vi "GitLoad.vi"(7 "Viewer?":bool, 8 "error in (no error)":errorcluster, 9 "Directory":path=path "", 10 "LoadThisHash":string, 11 "Git exec":string="git") -> (0 "error out":errorcluster, 1 "Directory out":path, 2 "Save Cluster":T1={"Version"="", "Devices"=[], "Select Layout"=0, "Layout:Strings And Values []"=[], "User defined functions"="-- -------------------------------------------------------------------------------------------\n-- The following functions are part of the \"standard load\" of functions and should not be messed with\n-- They are here for reference only.\n-- Please add any user functions above this comment\n-- -------------------------------------------------------------------------------------------\n\n-- Creates a linear ramp from A to B\nfunction LineRamp(f, Initial, Final)\n    return (1-f)*Initial + f*Final;\nend\n\n-- Creates an exponential ramp from A to B\nfunction ExpRamp(t, a, b, tau)\n   return (b - a*exp(tMax / tau) + (a-b)*exp(t/tau))/ ( 1 - exp(tMax / tau) );\nend\n\n-- Creates a sinewave\nfunction SinRamp(t,Offset,A,Freq, Phase)\n    return Offset + A * sin(2*pi*Freq*t + Phase)\nend\n\n-- Creates a blackman pulse\nfunction Blackman(f, Offset, A)\n    return Offset +  A*sqrt(0.5*cos(3.1415*(2*f-1))+0.08*cos(2*pi*(2*f-1))+0.42);\nend\n\n-- Creates a half-gauss ramp\nfunction HalfGaussRamp(t, a, b, Width)\n    local y;\n    y = exp(-(tMax^2)/Width^2);\n    y = (a -  b*y)/(1-y)  +  ((b-a)/(1-y))*exp(-((t-tMax)^2)/Width^2);\n    return y;\nend\n\n-- Creates an \"O'Hara\" ramp from A to B, for dipole evaporation\nfunction EvapRamp(t, a, b, tau)\n   local y;\n  y = log(a/b) / log(1+tMax/tau);\n  y = a * (1+t/tau)^(-y);\n  return y;\nend\n", "VariableManager"=refnum} {"Select Layout" items=["Default"]}, 3 "Git exec out":string, 4 "Loaded Description":string, 5 "User Cancelled":bool, 6 "Loaded Commit Info":T3)   [LabVIEW 2013]
uses:
  GitCommitCluster/CommitCluster.ctl
  TypeDefs/SaveCluster.ctl
  VariableManagerCodes/VariableManager/VariableManager.lvclass
  DeviceVIs/Device/Device.lvclass
  <vilib>/Utility/miscctls.llb/LVStringsAndValuesArrayTypeDef_I32.ctl
  <vilib>/Utility/miscctls.llb/LVPointTypeDef.ctl
  <vilib>/Utility/error.llb/DialogType.ctl
  <vilib>/Utility/miscctls.llb/LVRowAndColumnUnsignedTypeDef.ctl
panel:
  in  "WhichLoad":enum32{"Simple", "Filter"}(tab)
  in  "LoadSimple":bool
  in  "Page":u32=1 caption="Page (of 3)" min=1 max=3 step=1
  in  "SimpleProcedure":i32(listbox) caption="Pick a Procedure"
  in  "Cancel Button":bool
  in  "ToFilter":bool
  in  "CaseSensitive?":bool
  in  "MatchAll?":bool
  in  "Patterns":string[][](table)
  in  "AuthorList":i32[](listbox)
  out "Number Matched":i32
  in  "ApplyFilter":bool
  in  "AfterFilter":timestamp format="%<%H:%M:%S\n%Y/%m/%d>T"
  in  "BeforeFilter":timestamp format="%<%H:%M:%S\n%Y/%m/%d>T"
  in  "AfterDate?":bool
  in  "HashFilter":u64 format="%x"
  in  "Description?":bool
  in  "Author?":bool
  in  "BeforeDate?":bool
  in  "Hash?":bool
  in  "Cancel Button 2":bool
  in  "LoadFiltered":bool
  in  "ToSimple":bool
  in  "FilterProcedure":i32(listbox) caption="Pick a Procedure"
  # "Note: Sorting only affects entries on this page"
  # "(Uses grep-style expressions)"
  # "These are commit dates, which may be different from the \"date\" column."
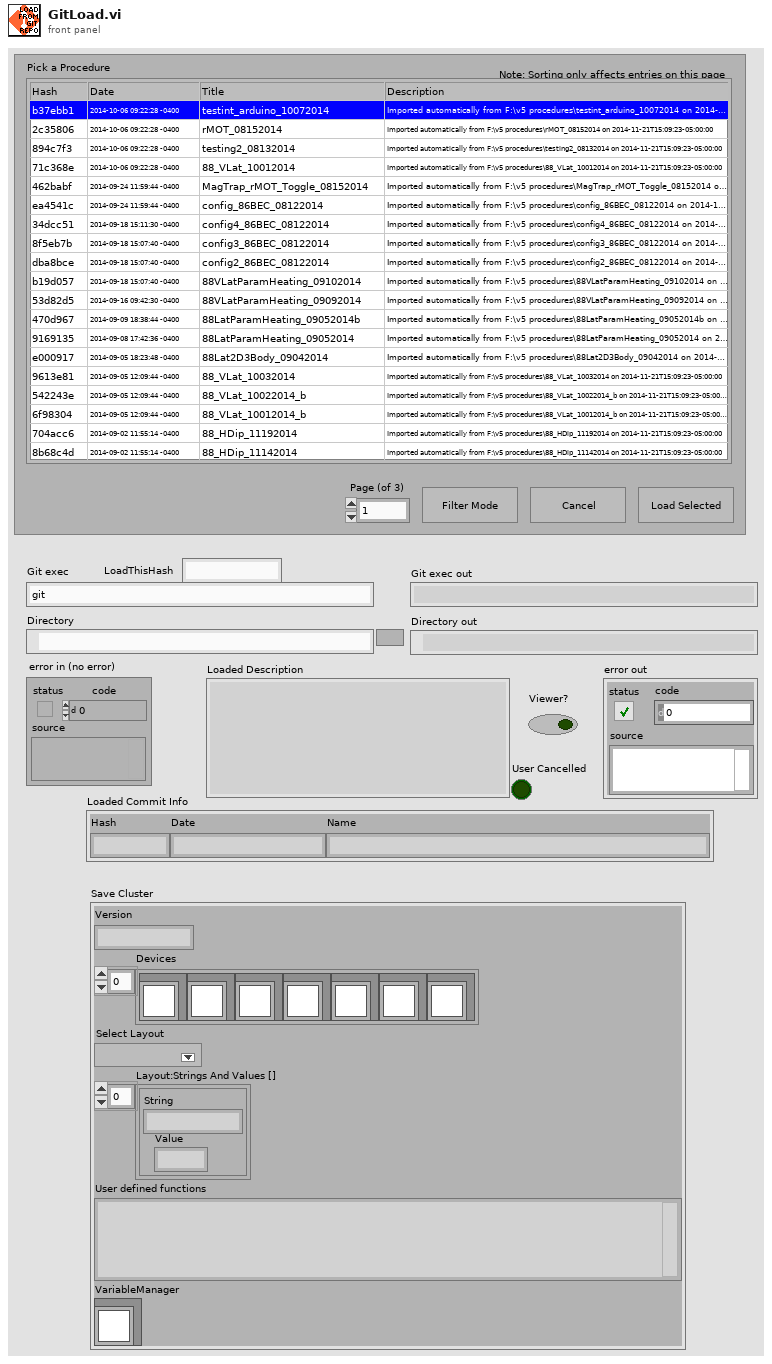
[diagram p1: front panel]
types:
  T1 = typedef "SaveCluster.ctl" = cluster{"Version":string, "Devices":refnum<class "Device.lvclass">[], "Select Layout":i32, "Layout:Strings And Values []":T2, "User defined functions":string, "VariableManager":refnum<class "VariableManager.lvclass">}
  T2 = typedef "LVStringsAndValuesArrayTypeDef_I32.ctl" = cluster{"String":string, "Value":i32}[]
  T3 = typedef "CommitCluster.ctl" = cluster{"Hash":string, "Date":string, "Name":string}
  T4 = typedef "DialogType.ctl" = u16
  T5 = typedef "LVPointTypeDef.ctl" = cluster{"Horizontal":i16, "Vertical":i16}
  T6 = typedef "LVRowAndColumnUnsignedTypeDef.ctl" = cluster{"Row":u32, "Column":u32}
  T7 = cluster{"Hash?":bool, "HashFilter":u64, "Description?":bool, "DescTitleFilters":string[], "MatchAll?":bool, "AfterDate?":bool, "AfterFilter":timestamp, "BeforeDate?":bool, "BeforeFilter":timestamp, "Author?":bool, "AuthorList":string[], "SelectedAuthors":i32[], "CaseSensitive?":bool}
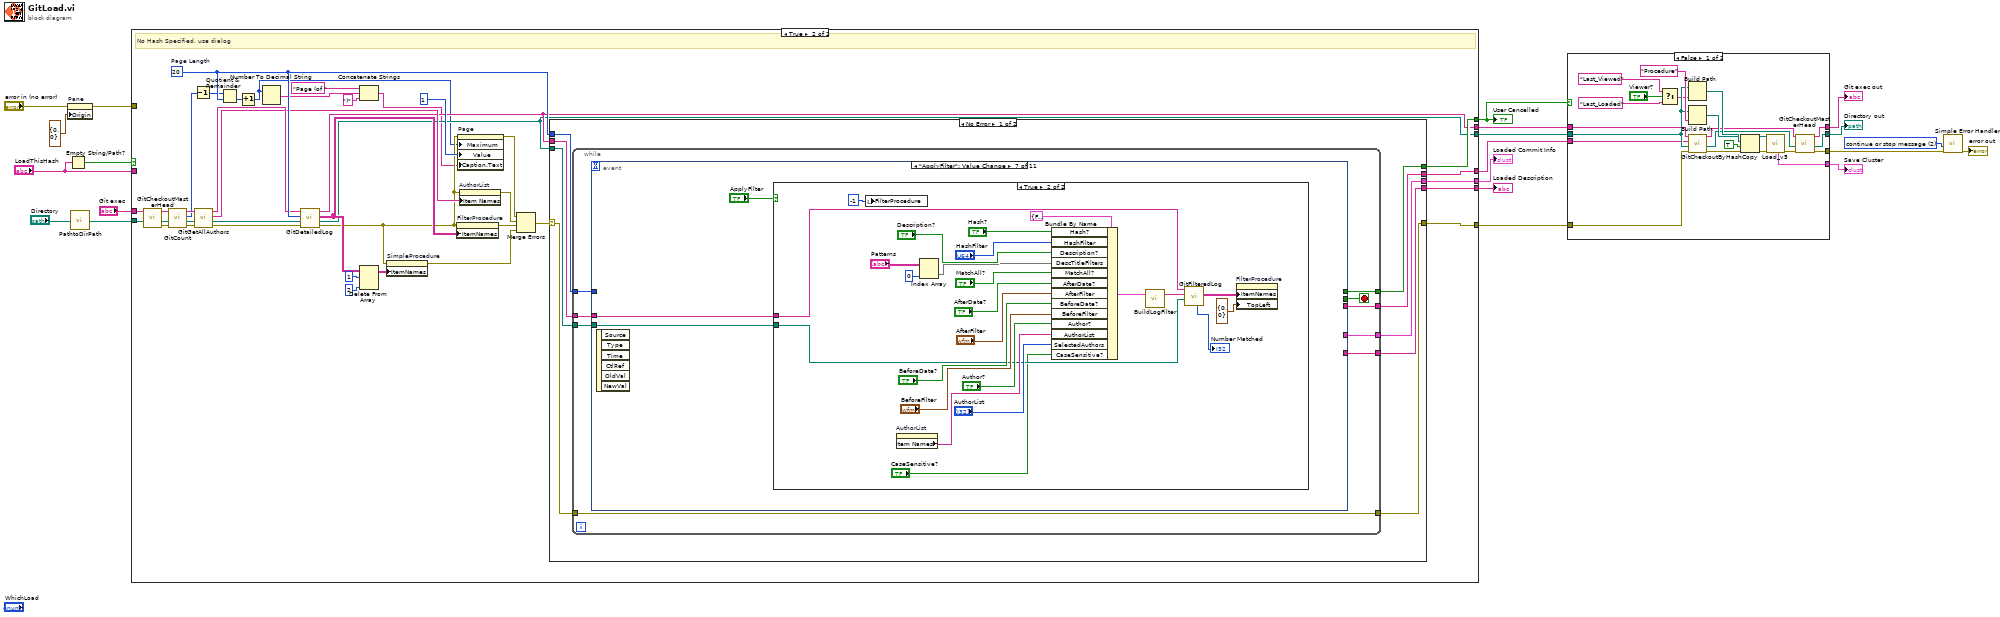
[diagram p0: block diagram]
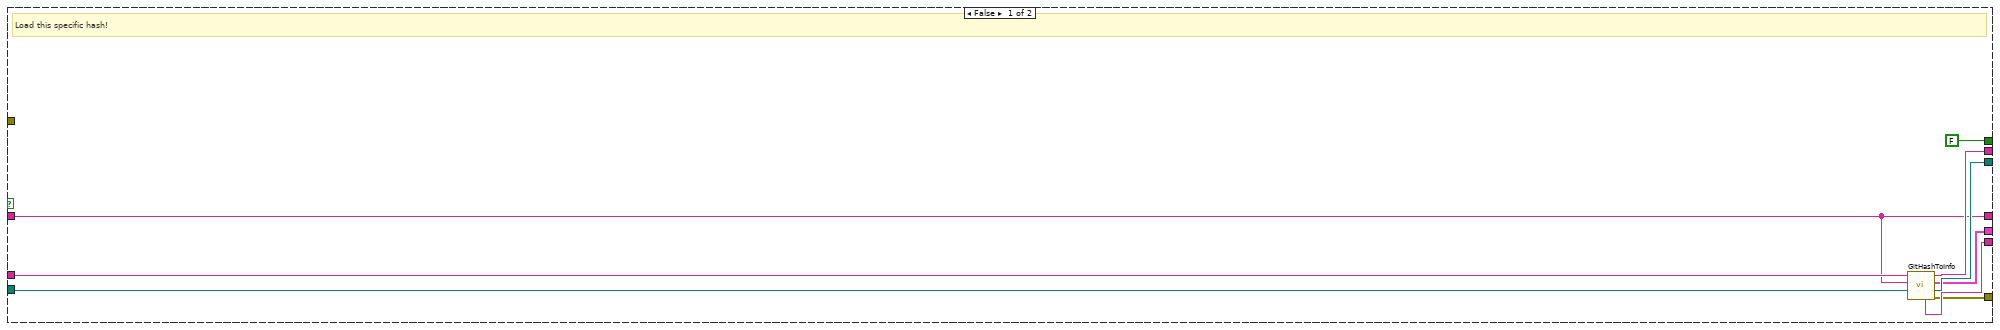
[diagram p2: hidden frame]
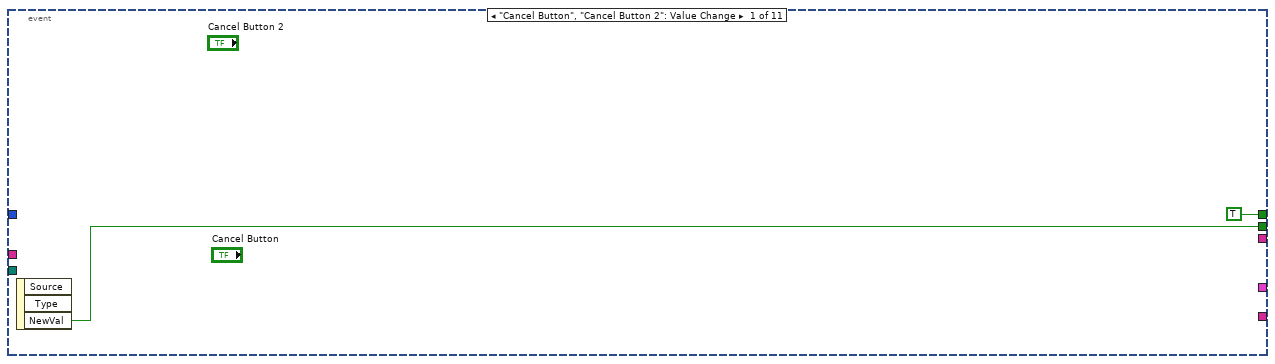
[diagram p3: hidden frame]
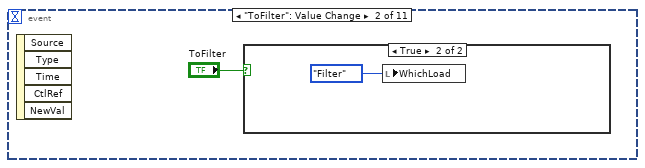
[diagram p4: hidden frame]
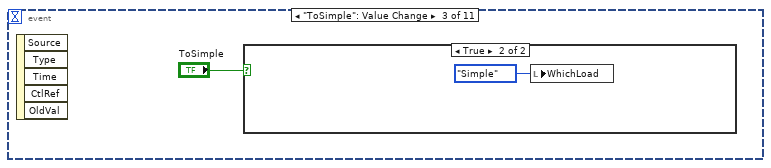
[diagram p6: hidden frame]
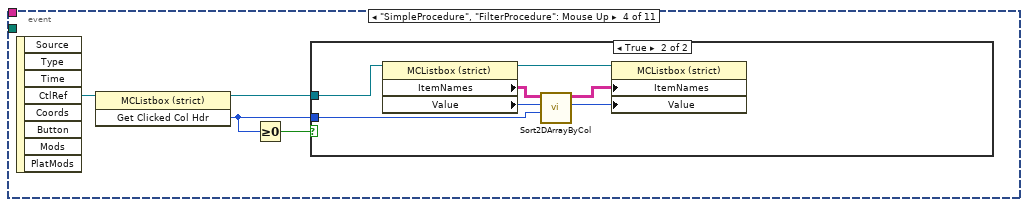
[diagram p8: hidden frame]
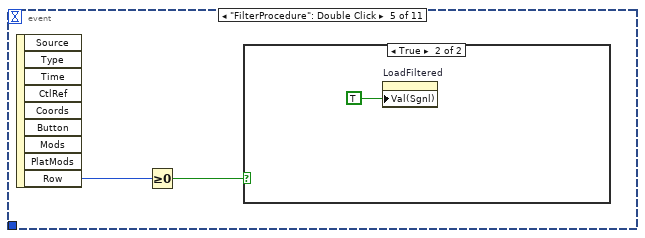
[diagram p10: hidden frame]
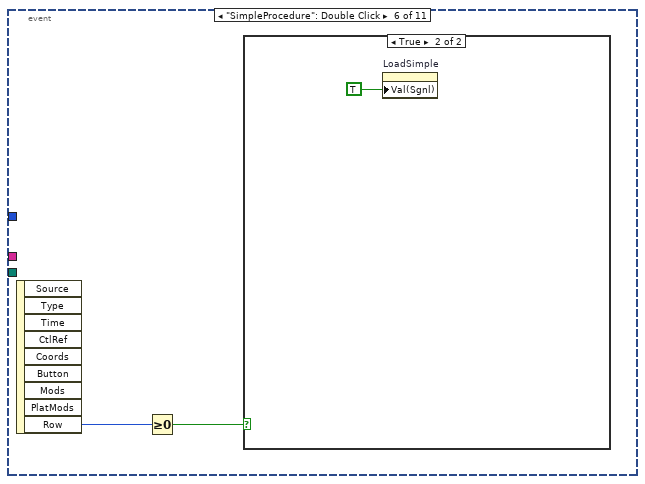
[diagram p12: hidden frame]
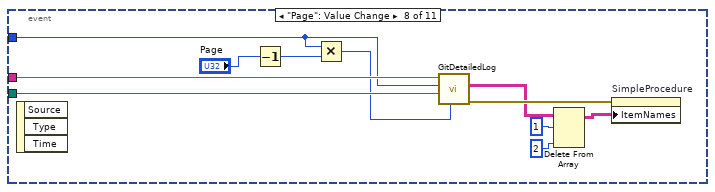
[diagram p15: hidden frame]
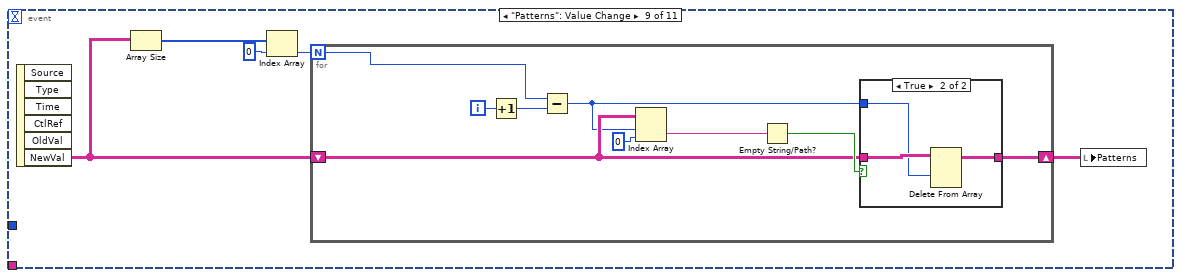
[diagram p16: hidden frame]
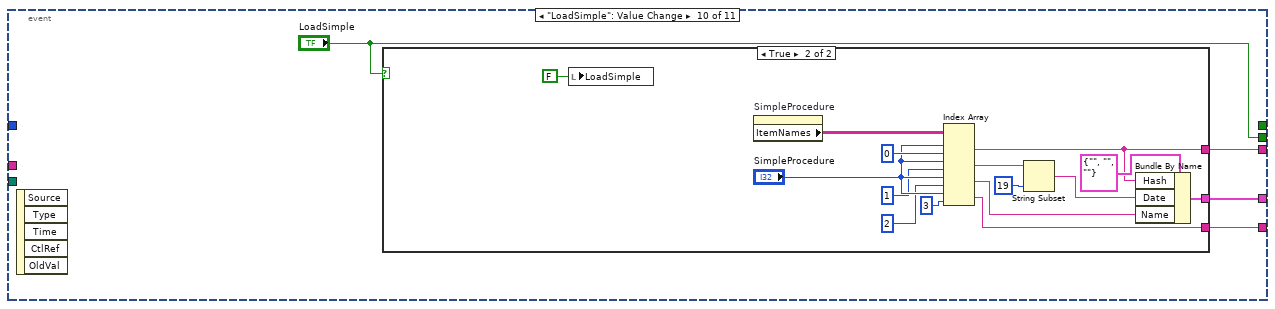
[diagram p18: hidden frame]
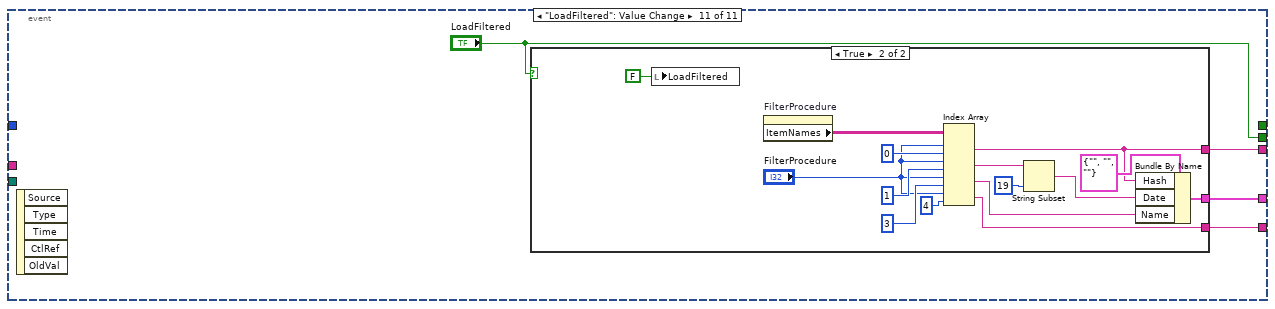
[diagram p20: hidden frame]
diagram:
  w3 = T4 2 items=["no dialog", "OK message", "continue or stop message", "OK message + warnings", "continue/stop + warnings"] ("type of dialog (OK msg:1)")
  n1 = property on="Pane" class="Pane"(error in="error in (no error)", "Origin"=T5 {"Horizontal"=0, "Vertical"=0}) -> (error out=w4:errorcluster)  [unwired: 1 in, 1 out]
  n2 = Empty String/Path?(string/path="LoadThisHash") -> (empty?=w6:bool)
  n3 = call "PathtoDirPath.vi"("Path"="Directory") -> ("Path out"=w15:path)
  n4 = case shown="True" w6 {
    tunnel: [w22 w56] -> w21
    tunnel: [FALSE w55] -> w20
    tunnel: [w28 w54] -> w19
    tunnel: [w29 w53] -> w18
    tunnel: "Git exec" -> [w27 w49]
    tunnel: w15 -> [w26 w48]
    tunnel: [w25 w47] -> w12
    tunnel: [w24 w46] -> w11
    tunnel: [w23 w39] -> w10
    tunnel: "LoadThisHash" -> [w22 _]
    tunnel: w4 -> [_ _]
    frame False {
      # "Load this specific hash!"
      n5 = call "GitHashToInfo.vi"("Directory"=w26, "Hash"=w22, "Git exec"=w27) -> ("error out"=w23:errorcluster, "Directory out"=w29:path, "Commit Info"=w25:T3, "Git exec out"=w28:string, "Description"=w24:string)  [unwired: 4 in]
    }
    frame True {
      w64 = 20  # Page Length
      # "No Hash Specified, use dialog"
      n6 = call "GitCheckoutMasterHead.vi"("File"=w48, "Git exec"=w49) -> ("error out"=w52:errorcluster, "File out"=w51:path, "Git exec out"=w50:string)  [unwired: 6 in, 1 out]
      n7 = call "GitCount.vi"("error in (no error)"=w52, "Directory"=w51, "Git exec"=w50) -> ("error out"=w59:errorcluster, "Directory out"=w60:path, "Count"=w37:u32, "Git exec out"=w62:string)  [unwired: 5 in]
      n8 = Decrement(x=w37) -> (x-1=w36:u32)
      n9 = call "GitGetAllAuthors.vi"("error in (no error)"=w59, "Directory"=w60, "Git exec"=w62) -> ("error out"=w45:errorcluster, "Directory out"=w58:path, "Author Array"=w57:string[], "Git exec out"=w61:string)  [unwired: 5 in]
      n10 = Quotient & Remainder(x=w36, y=w64) -> (floor(x/y)=w65:u32)  [unwired: 1 out]
      n11 = Increment(x=w65) -> (x+1=w31:u32)
      n12 = Number To Decimal String(number=w31) -> (decimal integer string=w32:string)  [unwired: 1 in]
      n13 = call "GitDetailedLog.vi"("error in (no error)"=w45, "Directory"=w58, "Number"=w64, "Git exec"=w61) -> ("error out"=w44:errorcluster, "Directory out"=w53:path, "Detail Array"=w63:string[][], "Git exec out"=w54:string)  [unwired: 4 in]
      n14 = Delete From Array(array=w63, length=1, index (col)=2 ("disabled index (col)")) -> (array with subset deleted=w69:string[][])  [unwired: 1 in, 1 out]
      n15 = Concatenate Strings("Page (of " ("string"), w32, ")" ("string")) -> (w33:string)
      n16 = property on="SimpleProcedure" class="MCListbox (strict)"(error in=w44, "ItemNames"=w69) -> (error out=w40:errorcluster)  [unwired: 1 in, 1 out]
      n17 = property on="FilterProcedure" class="MCListbox (strict)"(error in=w44, "ItemNames"=w63) -> (error out=w41:errorcluster)  [unwired: 1 in, 1 out]
      n18 = property on="Page" class="DigNum (strict)"(error in=w44, "Maximum"=w31, "Value"=u32 1 ("Page"), "Caption.Text"=w33) -> (error out=w43:errorcluster)  [unwired: 1 in, 1 out]
      n19 = property on="AuthorList" class="LstBox (strict)"(error in=w44, "Item Names"=w57) -> (error out=w42:errorcluster)  [unwired: 1 in, 1 out]
      n20 = Merge Errors(w43, w42, w41, w40) -> (w38:errorcluster)
      n21 = case shown="No Error" w38 {
        selector: w38 -> [w70 w205]
        tunnel: w64 -> [w78 _]
        tunnel: [w77 _] -> w56
        tunnel: [w76 TRUE] -> w55
        tunnel: w54 -> [w75 _]
        tunnel: w53 -> [w74 _]
        tunnel: [w73 _] -> w47
        tunnel: [w72 _] -> w46
        tunnel: [w71 w205] -> w39
        frame No Error {
          n22 = while {
            tunnel: w75 -> [w86]
            tunnel: w74 -> [w85]
            tunnel: w78 -> [w84]
            tunnel: [w83] -> w76
            tunnel: [w82] -> w77
            tunnel: [w81] -> w73
            tunnel: [w80] -> w72
            tunnel: w70 -> [w79]
            tunnel: [w79] -> w71
            stop <- w87 stop-if-true
            n23 = event shown="[6] \"ApplyFilter\": Value Change" {
              selector: _ -> [_ _ _ _ _ _ _ _ _ _ _]
              dyn-events: _ -> [_ _ _ _ _ _ _ _ _ _ _]
              timeout: _ -> [_ _ _ _ _ _ _ _ _ _ _]
              tunnel: [w88 _ _ _ _ _ _ _ _ "LoadSimple" "LoadFiltered"] -> w87
              tunnel: w86 -> [_ _ _ _ _ _ w112 w143 _ _ _]
              tunnel: w85 -> [_ _ _ _ _ _ w111 w142 _ _ _]
              tunnel: w84 -> [_ _ _ _ _ _ _ w141 _ _ _]
              tunnel: [TRUE _ _ _ _ _ _ _ _ _ _] -> w83
              tunnel: [_ _ _ _ _ _ _ _ _ w169 w189] -> w82
              tunnel: [_ _ _ _ _ _ _ _ _ w168 w186] -> w81
              tunnel: [_ _ _ _ _ _ _ _ _ w167 w187] -> w80
              event "Cancel Button", "Cancel Button 2": Value Change {
                n24 = event-data() -> ("NewVal"=w88:bool)  [unwired: 1 in, 2 out]
              }
              event "ToFilter": Value Change {
                n25 = event-data() -> ()  [unwired: 1 in, 5 out]
                n26 = case shown="True" "ToFilter" {
                  frame False {
                  }
                  frame True {
                    n27 = local write "WhichLoad"(enum32{"Simple", "Filter"}."Filter" ("WhichLoad")) -> ()
                  }
                }
              }
              event "ToSimple": Value Change {
                n28 = event-data() -> ()  [unwired: 1 in, 5 out]
                n29 = case shown="True" "ToSimple" {
                  frame False {
                  }
                  frame True {
                    n30 = local write "WhichLoad"(enum32{"Simple", "Filter"}."Simple" ("WhichLoad")) -> ()
                  }
                }
              }
              event "SimpleProcedure", "FilterProcedure": Mouse Up {
                n31 = event-data() -> ("CtlRef"=w95:refnum<vi>)  [unwired: 1 in, 7 out]
                n32 = invoke on="Invoke Node" class="MCListbox (strict)" method="Get Clicked Col Hdr"(reference=w95) -> (reference out=w94:refnum<vi>, "Get Clicked Column Header"=w96:i32)  [unwired: 2 in, 1 out]
                n33 = Greater Or Equal To 0?(x=w96) -> (x >= 0?=w97:bool)
                n34 = case shown="True" w97 {
                  tunnel: w96 -> [_ w104]
                  tunnel: w94 -> [_ w101]
                  frame False {
                  }
                  frame True {
                    n35 = property on="Property Node" class="MCListbox (strict)"(reference=w101) -> (reference out=w100:refnum<vi>, "ItemNames"=w103:string[][], "Value"=w98:i32)  [unwired: 1 in, 1 out]
                    n36 = call "Sort2DArrayByCol.vi"("Sort Column"=w104, "Current Selected Row"=w98, "ItemNames"=w103) -> ("Sorted Selected Row"=w99:i32, "Reversed 2D Array"=w102:string[][])  [unwired: 7 in]
                    n37 = property on="Property Node" class="MCListbox (strict)"(reference=w100, "ItemNames"=w102, "Value"=w99) -> ()  [unwired: 1 in, 2 out]
                  }
                }
              }
              event "FilterProcedure": Double Click {
                n38 = event-data() -> ("Row"=w106:i32)  [unwired: 1 in, 8 out]
                n39 = Greater Or Equal To 0?(x=w106) -> (x >= 0?=w105:bool)
                n40 = case shown="True" w105 {
                  frame False {
                  }
                  frame True {
                    n41 = property on="LoadFiltered" class="Bool (strict)"("Val(Sgnl)"=TRUE) -> ()  [unwired: 2 in, 2 out]
                  }
                }
              }
              event "SimpleProcedure": Double Click {
                n42 = event-data() -> ("Row"=w109:i32)  [unwired: 1 in, 8 out]
                n43 = Greater Or Equal To 0?(x=w109) -> (x >= 0?=w108:bool)
                n44 = case shown="True" w108 {
                  frame False {
                  }
                  frame True {
                    n45 = property on="LoadSimple" class="Bool (strict)"("Val(Sgnl)"=TRUE) -> ()  [unwired: 2 in, 2 out]
                  }
                }
              }
              event "ApplyFilter": Value Change {
                n46 = event-data() -> ()  [unwired: 1 in, 6 out]
                n47 = case shown="True" "ApplyFilter" {
                  tunnel: w112 -> [_ w125]
                  tunnel: w111 -> [_ w124]
                  frame False {
                  }
                  frame True {
                    n48 = local write "FilterProcedure"(-1 ("FilterProcedure")) -> ()
                    n49 = property on="AuthorList" class="LstBox (strict)"() -> ("Item Names"=w128:string[])  [unwired: 2 in, 2 out]
                    n50 = Index Array(array="Patterns", index (col)=0 ("disabled index (col)")) -> (element=w118:string[])  [unwired: 1 in]
                    n51 = Bundle By Name(cluster=T7 {"Hash?"=FALSE, "HashFilter"=0, "Description?"=FALSE, "DescTitleFilters"=[], "MatchAll?"=FALSE, "AfterDate?"=FALSE, "AfterFilter"=timestamp(0 s since 1904-01-01), "BeforeDate?"=FALSE, "BeforeFilter"=timestamp(0 s since 1904-01-01), "Author?"=FALSE, "AuthorList"=[], "SelectedAuthors"=[], "CaseSensitive?"=FALSE} ("FilterContents"), "Hash?"="Hash?", "HashFilter"="HashFilter", "Description?"="Description?", "DescTitleFilters"=w118, "MatchAll?"="MatchAll?", "AfterDate?"="AfterDate?", "AfterFilter"="AfterFilter", "BeforeDate?"="BeforeDate?", "BeforeFilter"="BeforeFilter", "Author?"="Author?", "AuthorList"=w128, "SelectedAuthors"="AuthorList", "CaseSensitive?"="CaseSensitive?") -> (w116:T7)
                    n52 = call "BuildLogFilter.vi"("FilterContents"=w116) -> ("FilterString"=w126:string)  [unwired: 2 in]
                    n53 = call "GitFilteredLog.vi"("Directory"=w124, "Filter"=w126, "Git exec"=w125) -> ("Detail Array"=w123:string[][], "Number Matched"=→"Number Matched":i32)  [unwired: 4 in, 3 out]
                    n54 = property on="FilterProcedure" class="MCListbox (strict)"("ItemNames"=w123, "TopLeft"=T6 {"Row"=0, "Column"=0} ("Top Left Visible Cell")) -> ()  [unwired: 2 in, 2 out]
                  }
                }
              }
              event "Page": Value Change {
                n55 = event-data() -> ()  [unwired: 1 in, 3 out]
                n56 = Decrement(x="Page") -> (x-1=w138:u32)
                n57 = Multiply(x=w141, y=w138) -> (x*y=w140:u32)
                n58 = call "GitDetailedLog.vi"("skip"=w140, "Directory"=w142, "Number"=w141, "Git exec"=w143) -> ("error out"=w148:errorcluster, "Detail Array"=w144:string[][])  [unwired: 4 in, 2 out]
                n59 = Delete From Array(array=w144, length=1, index (col)=2 ("disabled index (col)")) -> (array with subset deleted=w145:string[][])  [unwired: 1 in, 1 out]
                n60 = property on="SimpleProcedure" class="MCListbox (strict)"(error in=w148, "ItemNames"=w145) -> ()  [unwired: 1 in, 2 out]
              }
              event "Patterns": Value Change {
                n61 = event-data() -> ("NewVal"=w150:string[][])  [unwired: 1 in, 5 out]
                n62 = Array Size(array=w150) -> (size(s)=w153:i32[])
                n63 = Index Array(array=w153, index=0) -> (element=w151:i32)
                n64 = for {
                  N: w151 -> [w162]
                  shift-right: [w155] -> w149
                  shift-left: w150 -> [w156]
                  i -> [w161]
                  n65 = Increment(x=w161) -> (x+1=w160:i32)
                  n66 = Subtract(x=w162, y=w160) -> (x-y=w154:i32)
                  n67 = Index Array(array=w156, index (row)=w154, index (col)=0 ("disabled index (col)")) -> (element=w158:string)
                  n68 = Empty String/Path?(string/path=w158) -> (empty?=w157:bool)
                  n69 = case shown="True" w157 {
                    tunnel: w156 -> [w163 w166]
                    tunnel: [w163 w165] -> w155
                    tunnel: w154 -> [_ w164]
                    frame False {
                    }
                    frame True {
                      n70 = Delete From Array(array=w166, index (row)=w164) -> (array with subset deleted=w165:string[][])  [unwired: 2 in, 1 out]
                    }
                  }
                }
                n71 = local write "Patterns"(w149) -> ()
              }
              event "LoadSimple": Value Change {
                n72 = event-data() -> ()  [unwired: 1 in, 5 out]
                n73 = case shown="True" "LoadSimple" {
                  tunnel: [_ w181] -> w169
                  tunnel: [_ w182] -> w168
                  tunnel: [_ w176] -> w167
                  frame False {
                  }
                  frame True {
                    n74 = local write "LoadSimple"(FALSE ("LoadSimple")) -> ()
                    n75 = property on="SimpleProcedure" class="MCListbox (strict)"() -> ("ItemNames"=w185:string[][])  [unwired: 2 in, 2 out]
                    n76 = Index Array(array=w185, index (row) #1="SimpleProcedure", index (col) #1=0 ("index"), index (row) #2="SimpleProcedure", index (col) #2=1 ("disabled index (col)"), index (row) #3="SimpleProcedure", index (col) #3=2 ("disabled index (col)"), index (row) #4="SimpleProcedure", index (col) #4=3 ("disabled index (col)")) -> (element #1=w181:string, element #2=w173:string, element #3=w175:string, element #4=w176:string)
                    n77 = String Subset(string=w173, length (rest)=19 ("length (rest)")) -> (substring=w174:string)  [unwired: 1 in]
                    n78 = Bundle By Name(cluster=T3 {"Hash"="", "Date"="", "Name"=""} ("Commit"), "Hash"=w181, "Date"=w174, "Name"=w175) -> (w182:T3)
                  }
                }
              }
              event "LoadFiltered": Value Change {
                n79 = event-data() -> ()  [unwired: 1 in, 5 out]
                n80 = case shown="True" "LoadFiltered" {
                  tunnel: [_ w197] -> w189
                  tunnel: [_ w195] -> w187
                  tunnel: [_ w194] -> w186
                  frame False {
                  }
                  frame True {
                    n81 = local write "LoadFiltered"(FALSE ("LoadFiltered")) -> ()
                    n82 = property on="FilterProcedure" class="MCListbox (strict)"() -> ("ItemNames"=w204:string[][])  [unwired: 2 in, 2 out]
                    n83 = Index Array(array=w204, index (row) #1="FilterProcedure", index (col) #1=0 ("index"), index (row) #2="FilterProcedure", index (col) #2=1 ("disabled index (col)"), index (row) #3="FilterProcedure", index (col) #3=3 ("disabled index (col)"), index (row) #4="FilterProcedure", index (col) #4=4 ("disabled index (col)")) -> (element #1=w197:string, element #2=w192:string, element #3=w196:string, element #4=w195:string)
                    n84 = String Subset(string=w192, length (rest)=19 ("length (rest)")) -> (substring=w191:string)  [unwired: 1 in]
                    n85 = Bundle By Name(cluster=T3 {"Hash"="", "Date"="", "Name"=""} ("Commit"), "Hash"=w197, "Date"=w191, "Name"=w196) -> (w194:T3)
                  }
                }
              }
            }
          }
        }
        frame Error {
        }
      }
    }
  }
  "User Cancelled" <- w20
  "Loaded Description" <- w11
  "Loaded Commit Info" <- w12
  n86 = case shown="False" w20 {
    tunnel: w21 -> [w219 _]
    tunnel: w18 -> [w226 w231]
    tunnel: w19 -> [w228 w230]
    tunnel: [w217 w230] -> w14
    tunnel: [w216 w231] -> w13
    tunnel: [w211 w229] -> w2
    tunnel: w10 -> [w218 w229]
    tunnel: [w213 _] -> w9
    frame False {
      n87 = Select(t="Last_Viewed", s="Viewer?", f="Last_Loaded" ("name or relative path")) -> (s? t:f=w208:string)
      n88 = Build Path(base path=w226, name or relative path=w208) -> (appended path=w225:path)
      n89 = Build Path(base path=w226, name or relative path="Procedure") -> (appended path=w224:path)
      n90 = call "GitCheckoutByHash.vi"("error in (no error)"=w218, "File"=w226, "Hash"=w219, "Git exec"=w228) -> ("error out"=w220:errorcluster, "File out"=w221:path, "Git exec out"=w222:string)  [unwired: 4 in, 1 out]
      n91 = Copy(8:w220, 9:TRUE ("overwrite (F)"), 10:w225, 11:w224) -> (0:w214:errorcluster, 3:w215:path)  [unwired: 1 in, 1 out]
      n92 = call "Load_v5.vi"("error in"=w214, "Path (open dialog)"=w215) -> ("error out"=w212:errorcluster, "Save Cluster"=w213:T1)  [unwired: 5 in, 3 out]
      n93 = call "GitCheckoutMasterHead.vi"("error in (no error)"=w212, "File"=w221, "Git exec"=w222) -> ("error out"=w211:errorcluster, "File out"=w216:path, "Git exec out"=w217:string)  [unwired: 5 in, 1 out]
    }
    frame True {
    }
  }
  "Git exec out" <- w14
  "Directory out" <- w13
  "Save Cluster" <- w9
  n94 = call <vilib>:"Simple Error Handler.vi"("type of dialog (OK msg:1)"=w3, "error in (no error)"=w2) -> ("error out"=→"error out":errorcluster)  [unwired: 3 in, 4 out]
